vi "Release.vi"(8 "error in (no error)":errorcluster, 11 "TriggerAction in":refnum<class "TriggerAction Q.lvclass">) -> (0 "error out":errorcluster, 3 "TriggerAction out":refnum<class "TriggerAction Q.lvclass">)   [LabVIEW 2016, in "TriggerAction Q.lvclass"]
uses:
  <userlib>/Common Components/TriggerAction Q/TriggerAction Q/TriggerAction Q.lvclass
  <userlib>/Common Components/TriggerAction Q/TriggerAction Q/TriggerAction Q.lvclass/TriggerAction Q.ctl
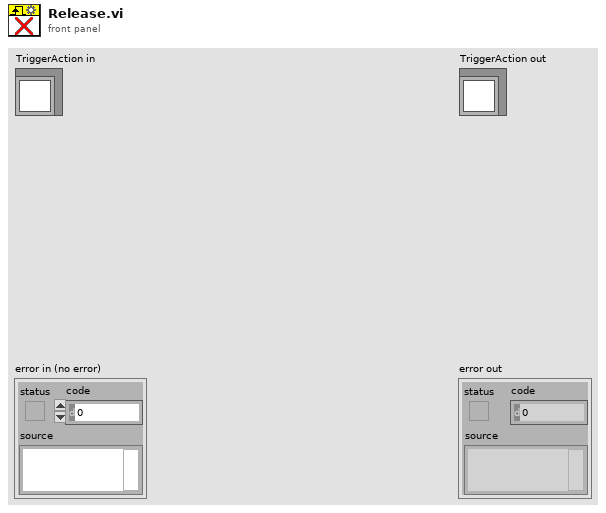
[diagram p1: front panel]
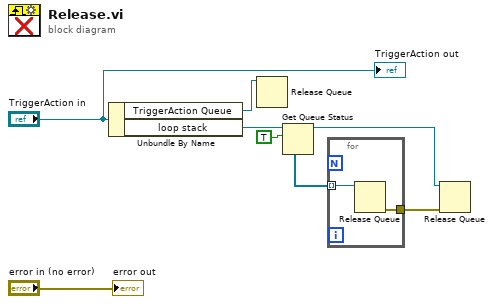
[diagram p0: block diagram]
diagram:
  n1 = Unbundle By Name("TriggerAction in") -> ("TriggerAction Queue"=w7:refnum<queue>, "loop stack"=w5:refnum<queue>)
  n2 = Release Queue(queue=w7) -> ()  [unwired: 2 in, 3 out]
  n3 = Get Queue Status(queue=w5, return elements? (F)=TRUE) -> (queue out=w2:refnum<queue>, elements=w3:refnum<queue>[])  [unwired: 1 in, 6 out]
  n4 = for {
    tunnel: w3 -> [w10] mode=indexing
    tunnel: [w9] -> w1
    n5 = Release Queue(queue=w10) -> (error out=w9:errorcluster)  [unwired: 2 in, 2 out]
  }
  n6 = Release Queue(queue=w2, error in (no error)=w1) -> ()  [unwired: 1 in, 3 out]
  "error out" <- "error in (no error)"
  "TriggerAction out" <- "TriggerAction in"
